vi "Send Core.vi"(6 "Severity Code (info)":T1=enum."info", 8 "Error In":errorcluster, 9 "Message Content":string, 10 "Message Tag":string, 11 "BNT_SLMsgLogger in":refnum<class "BNT_SLMsgLogger.lvclass">) -> (0 "Error Out":errorcluster, 3 "BNT_SLMsgLogger out":refnum<class "BNT_SLMsgLogger.lvclass">)   [LabVIEW 2019, in "BNT_SLMsgLogger.lvlib" / "BNT_SLMsgLogger.lvclass"]
doc: "Send mesage to message logger."
uses:
  BNT_SLMsgLogger.lvclass
  CSPP_Core/Libraries/Base/Severity.ctl
  BNT_SLMsgLogger.lvclass/BNT_SLMsgLogger.ctl
  <vilib>/Skyline/Message/NI Skyline Message.lvclass
  CSPP_Core/Libraries/Base/CSPP_Base.lvlib
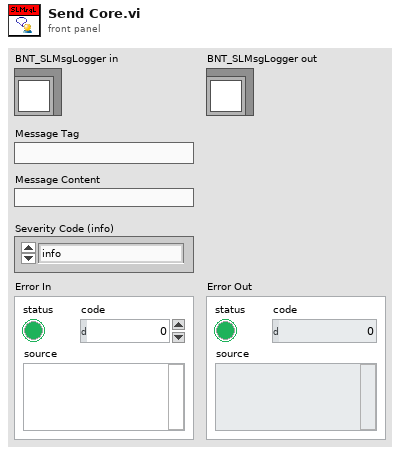
[diagram p1: front panel]
types:
  T1 = typedef "CSPP_Base.lvlib/Severity.ctl" = enum16{"emergency", "alert", "critical", "error", "warning", "notice", "info", "debug"}
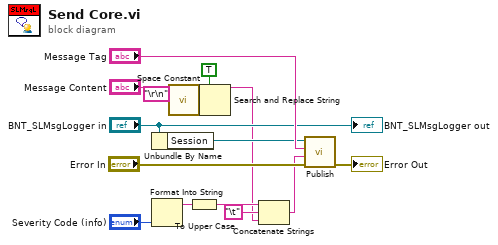
[diagram p0: block diagram]
diagram:
  n1 = Unbundle By Name("BNT_SLMsgLogger in") -> ("Session"=w13:refnum<class "NI Skyline Message.lvclass">)
  n2 = Format Into String("Severity Code (info)") -> (resulting string=w9:string)  [unwired: 3 in, 1 out]
  n3 = call <vilib>:"Space Constant.vi"() -> ("String"=w2:string)
  n4 = To Upper Case(1:w9) -> (0:w8:string)
  n5 = Search and Replace String(replace all?=TRUE ("replace all? (F)"), input string="Message Content", search string="\r\n", replace string=w2) -> (result string=w5:string)  [unwired: 4 in, 3 out]
  n6 = Concatenate Strings(w8, "\t", w5) -> (w7:string)
  n7 = call-dynamic "Publish.vi"("error in (no error)"="Error In", "message"=w7, "topic"="Message Tag", "message session in"=w13) -> ("error out"=→"Error Out":errorcluster)  [unwired: 6 in, 1 out]
  "BNT_SLMsgLogger out" <- "BNT_SLMsgLogger in"
